vi "TDC_errorHandler.vi"(8 "quTAU Return Code":i32, 11 "Error In":errorcluster) -> (3 "Error Out":errorcluster)   [LabVIEW 2011]
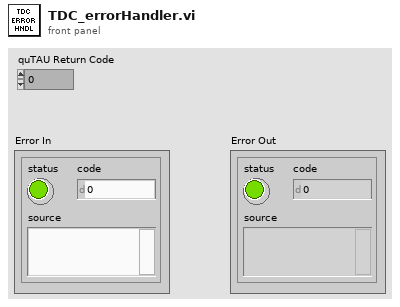
[diagram p1: front panel]
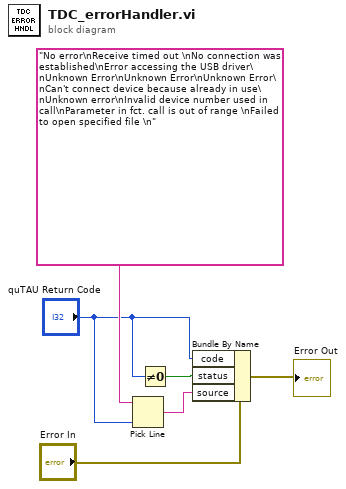
[diagram p0: block diagram]
diagram:
  n1 = Pick Line(multi-line string="No error\nReceive timed out \nNo connection was established\nError accessing the USB driver\nUnknown Error\nUnknown Error\nUnknown Error\nCan't connect device because already in use\nUnknown error\nInvalid device number used in call\nParameter in fct. call is out of range \nFailed to open specified file \n", line index="quTAU Return Code") -> (output string=w3:string)  [unwired: 1 in]
  n2 = Not Equal To 0?(x="quTAU Return Code") -> (x != 0?=w4:bool)
  n3 = Bundle By Name(cluster="Error In", "code"="quTAU Return Code", "status"=w4, "source"=w3) -> (→"Error Out":errorcluster)
